vi "DSDLL Initialize Virtual Channels.vi"(8 "error in":errorcluster, 11 "dsdll session":T1) -> (0 "error out":errorcluster, 1 "combined device name":string, 2 "channel names":string[](array[string]), 3 "dsdll session out":T1)   [LabVIEW 2018, in "DSDLL Virtual Digitizer.lvlib"]
doc: "Initializes dsdll virtual channels. In fact it just tests the capture device and the device stays closed untill call of 'Setup Virtual Channels'."
uses:
  DSDLL Virtual Digitizer.lvlib
  DSDLL Session.ctl
  dsdll source distribution/dsdll_instance.ctl
  dsdll source distribution/dsdll_device_record.ctl
  DSDLL Process Config.ctl
  DSDLL Data Packet.ctl
  dsdll source distribution/dsdll_format.ctl
  dsdll source distribution/dsdll_sample_format.ctl
  dsdll source distribution/dsdll.lvlib
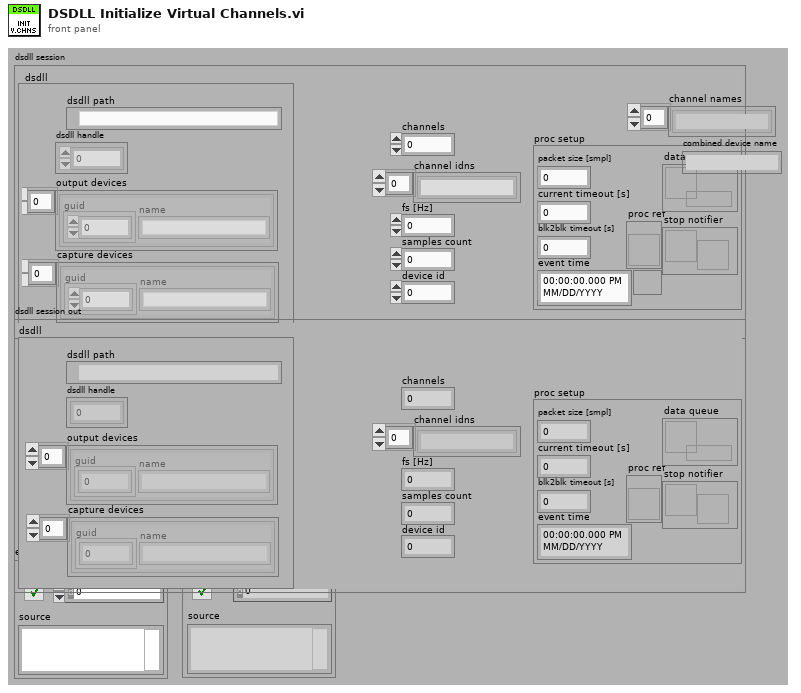
[diagram p1: front panel]
types:
  T1 = typedef "DSDLL Virtual Digitizer.lvlib/DSDLL Session.ctl" = cluster{"dsdll":T2, "channels":i32, "device id":i32, "channel idns":string[], "proc setup":T4, "samples count":i32, "fs [Hz]":dbl}
  T2 = typedef "dsdll.lvlib/dsdll_instance.ctl" = cluster{"dsdll path":path, "dsdll handle":u8[], "output devices":T3[], "capture devices":T3[]}
  T3 = typedef "dsdll.lvlib/dsdll_device_record.ctl" = cluster{"guid":u8[], "name":string}
  T4 = typedef "DSDLL Virtual Digitizer.lvlib/DSDLL Process Config.ctl" = cluster{"packet size [smpl]":i32, "current timeout [s]":dbl, "blk2blk timeout [s]":dbl, "event time":timestamp, "data queue":refnum<queue>, "stop notifier":refnum<notifier>, "proc ref":refnum<vi>}
  T5 = typedef "dsdll.lvlib/dsdll_sample_format.ctl" = enum16{"IEEE float 32", "PCM 16 bit"}
  T6 = typedef "dsdll.lvlib/dsdll_format.ctl" = cluster{"sample rate [Hz]":u32, "out channels":u16, "inp channels":u16, "format":T5}
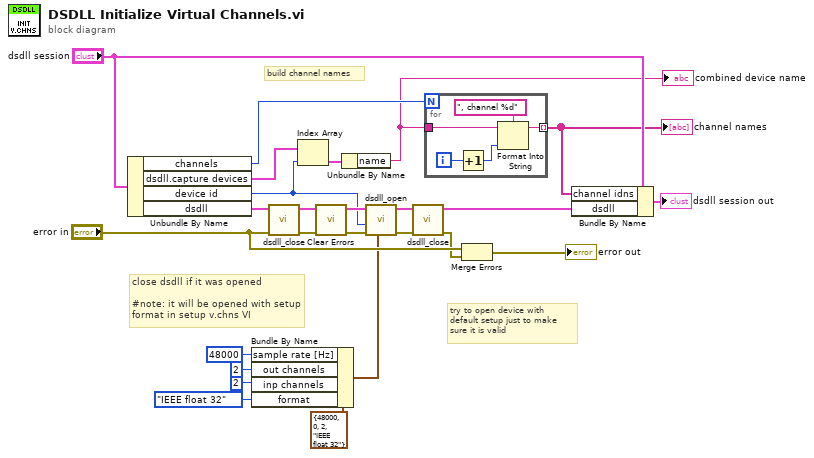
[diagram p0: block diagram]
diagram:
  # "build channel names"
  # "try to open device with\ndefault setup just to make\nsure it is valid"
  # "close dsdll if it was opened\n\n#note: it will be opened with setup\nformat in setup v.chns VI"
  n1 = Unbundle By Name("dsdll session") -> ("channels"=w9:i32, "dsdll.capture devices"=w12:T3[], "device id"=w11:i32, "dsdll"=w22:T2)
  n2 = Bundle By Name(cluster=T6 {"sample rate [Hz]"=48000, "out channels"=0, "inp channels"=2, "format"=enum."IEEE float 32"} ("format"), "sample rate [Hz]"=u32 48000, "out channels"=u16 2, "inp channels"=u16 2, "format"=dsdll_sample_format."IEEE float 32") -> (w5:T6)
  n3 = call "dsdll_close.vi"("error in"="error in", "dsdll instance in"=w22) -> ("error out"=w19:errorcluster, "dsdll instance out"=w15:T2)  [unwired: 8 in]
  n4 = Index Array(array=w12, index=w11) -> (element=w10:T3)
  n5 = call <vilib>:"Clear Errors.vi"("error in (no error)"=w19) -> ("error out"=w18:errorcluster)  [unwired: 5 in, 1 out]
  n6 = Unbundle By Name(w10) -> ("name"=w8:string)
  "combined device name" <- w8
  n7 = call "dsdll_open.vi"("format"=w5, "error in"=w18, "capture device id"=w11, "dsdll instance in"=w15) -> ("error out"=w17:errorcluster, "dsdll instance out"=w14:T2)  [unwired: 6 in]
  n8 = call "dsdll_close.vi"("error in"=w17, "dsdll instance in"=w14) -> ("error out"=w16:errorcluster, "dsdll instance out"=w13:T2)  [unwired: 8 in]
  n9 = for {
    N: w9 -> [_]
    tunnel: w8 -> [w29]
    tunnel: [w28] -> w7 mode=indexing
    i -> [w27]
    n10 = Increment(x=w27) -> (x+1=w26:i32)
    n11 = Format Into String(format string=", channel %d", initial string=w29, w26) -> (resulting string=w28:string)  [unwired: 1 in, 1 out]
  }
  "channel names" <- w7
  n12 = Merge Errors("error in", w16) -> (→"error out":errorcluster)
  n13 = Bundle By Name(cluster="dsdll session", "channel idns"=w7, "dsdll"=w13) -> (→"dsdll session out":T1)
